vi "dbltest.vi"(11 "Data In":dbl) -> (3 "Data Out":dbl)   [LabVIEW 2016]
doc: "Assert Component\nAssert Name: dbltest\nData Type: Double Float\nDeveloped by UKHornP\nEvaluation String: X = 10.000000\nDescription: blah"
uses:
  Core/Assert API Components/Failure Actions.ctl
  Core/Assert API Components/VI References.ctl
  Core/Assert API Components/Assert API Components.lvlib
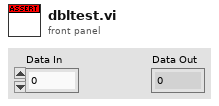
[diagram p1: front panel]
types:
  T1 = typedef "Assert API Components.lvlib/VI References.ctl" = cluster{"Calling VI Ref":refnum<vi>, "Assert VI Ref":refnum<vi>}
  T2 = typedef "Assert API Components.lvlib/Failure Actions.ctl" = enum16{"None", "Log To File", "Pause Execution", "Abort Execution"}
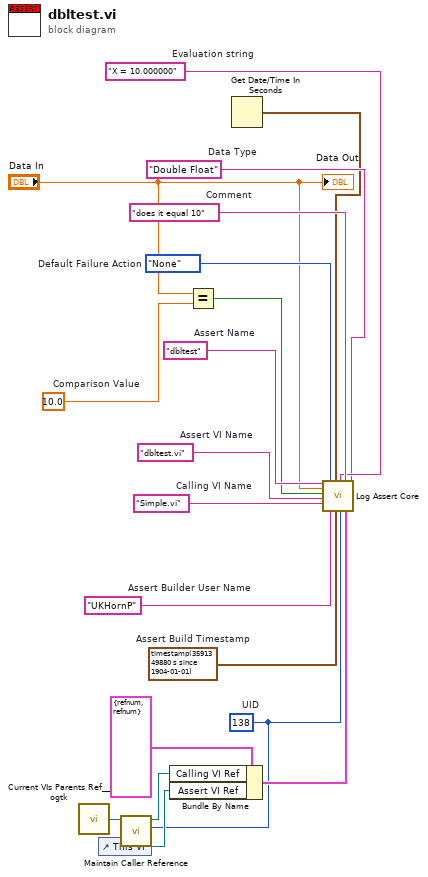
[diagram p0: block diagram]
diagram:
  w1 = 138  # UID
  w5 = "dbltest.vi"  # Assert VI Name
  w6 = "Simple.vi"  # Calling VI Name
  w7 = timestamp(3591349880.026634 s since 1904-01-01)  # Assert Build Timestamp
  w8 = "UKHornP"  # Assert Builder User Name
  w9 = "Double Float"  # Data Type
  w16 = "does it equal 10"  # Comment
  w13 = "X = 10.000000"  # Evaluation string
  w18 = Failure_Actions."None"  # Default Failure Action
  w19 = "dbltest"  # Assert Name
  w17 = 10.0  # Comparison Value
  n1 = call <userlib>:"Current VIs Parents Ref__ogtk.vi"() -> ("Calling VI's Reference"=w3:refnum<vi>)  [unwired: 2 in]
  n2 = control-ref of="This VI"() -> (w11:refnum<vi>)
  n3 = call "Maintain Caller Reference.vi"("UID"=w1, "VI in"=w3) -> ("VI out"=w2:refnum<vi>)  [unwired: 9 in]
  n4 = Bundle By Name(cluster=T1 {"Calling VI Ref"=refnum, "Assert VI Ref"=refnum} ("VI References"), "Calling VI Ref"=w2, "Assert VI Ref"=w11) -> (w10:T1)
  n5 = Equal?(x="Data In", y=w17) -> (x = y?=w14:bool)
  n6 = Get Date/Time In Seconds() -> (seconds since 1Jan1904=w4:timestamp)
  n7 = call "Log Assert Core.vi"("Assert Name"=w19, "Data Value"="Data In", "Status"=w14, "Assert VI Name"=w5, "Calling VI Name"=w6, "Failure Action"=w18, "Assert Builder User Name"=w8, "Last Update"=w4, "Assert Build Timestamp"=w7, "Evaluation String"=w13, "Assert VI UID"=w1, "Comment"=w16, "VI References"=w10, "Data Type"=w9) -> ()  [unwired: 6 in]
  "Data Out" <- "Data In"
